vi "CANOpen_Format dynamicSDO to String Array.vi"(7 "Display format":T1=enum."Decimal", 8 "error in (no error)":errorcluster, 11 "SDO Parameters":T2[](array[typedef]) {"Sub-Index (0)" format="%.0x"; "Object Index" format="%.0x"; "Block Data" format="%.0x"}) -> (0 "error out":errorcluster, 3 "Array":string[][](array[string]))   [LabVIEW 2013, in "CANOpen Addon Custom Device.lvlib"]
uses:
  CANOpen Addon Custom Device.lvlib
  Shared Code/CANOpen_SDO Settings.ctl
  CANOpen_SDO data format.ctl
panel:
  # "LSB"
  # "MSB"
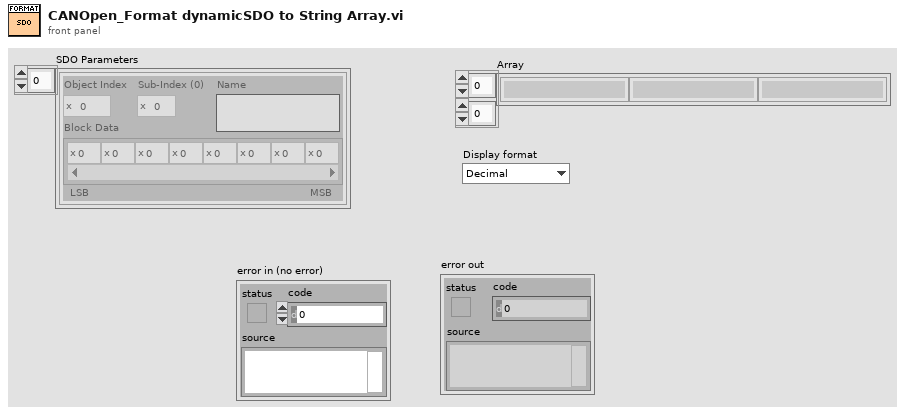
[diagram p1: front panel]
types:
  T1 = typedef "CANOpen Addon Custom Device.lvlib/CANOpen_SDO data format.ctl" = enum16{"Hexadecimal", "Decimal"}
  T2 = typedef "CANOpen Addon Custom Device.lvlib/CANOpen_SDO Settings.ctl" = cluster{"Object Index":u16, "Sub-Index (0)":u8, "Block Data":u8[], "Name":string}
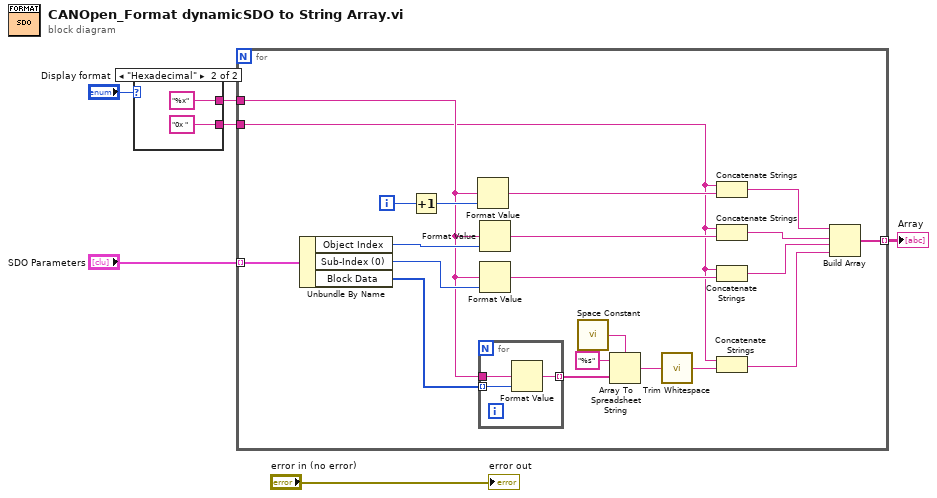
[diagram p0: block diagram]
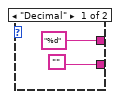
[diagram p2: hidden frame]
diagram:
  n1 = case shown="\"Hexadecimal\"" "Display format" {
    tunnel: ["%d" "%x"] -> w5
    tunnel: ["" "0x "] -> w1
    frame "Decimal" {
    }
    frame "Hexadecimal" {
    }
  }
  n2 = for {
    tunnel: "SDO Parameters" -> [w31] mode=indexing
    tunnel: w5 -> [w20]
    tunnel: [w23] -> w3 mode=indexing
    tunnel: w1 -> [w15]
    i -> [w22]
    n3 = Unbundle By Name(w31) -> ("Object Index"=w28:u16, "Sub-Index (0)"=w29:u8, "Block Data"=w30:u8[])
    n4 = Increment(x=w22) -> (x+1=w21:i32)
    n5 = Format Value(format string=w20, value (0)=w21) -> (output string=w16:string)  [unwired: 1 in]
    n6 = for {
      tunnel: w30 -> [w34] mode=indexing
      tunnel: w20 -> [w33]
      tunnel: [w32] -> w27 mode=indexing
      n7 = Format Value(format string=w33, value (0)=w34) -> (output string=w32:string)  [unwired: 1 in]
    }
    n8 = Format Value(format string=w20, value (0)=w28) -> (output string=w17:string)  [unwired: 1 in]
    n9 = Format Value(format string=w20, value (0)=w29) -> (output string=w18:string)  [unwired: 1 in]
    n10 = call <vilib>:"Space Constant.vi"() -> ("String"=w25:string)
    n11 = Array To Spreadsheet String(delimiter (Tab)=w25, array=w27, 3:"%s" ("format string")) -> (spreadsheet string=w24:string)
    n12 = call <vilib>:"Trim Whitespace.vi"("string"=w24) -> ("trimmed string"=w19:string)  [unwired: 1 in]
    n13 = Concatenate Strings(w15, w16) -> (w14:string)
    n14 = Concatenate Strings(w15, w17) -> (w13:string)
    n15 = Concatenate Strings(w15, w18) -> (w12:string)
    n16 = Concatenate Strings(w15, w19) -> (w11:string)
    n17 = Build Array(w14, w13, w12, w11) -> (w23:string[])
  }
  "Array" <- w3
  "error out" <- "error in (no error)"
